vi "Testvi.vi"() -> ()   [LabVIEW 2019]
uses:
  <vilib>/addons/control/pid/pid.llb/PID (DBL).vi
  <vilib>/addons/control/pid/NI_PID_pid.lvlib
panel:
  in  "process variable":dbl format="%.2f"
  in  "setpoint":dbl format="%.2f"
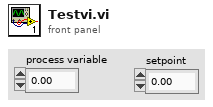
[diagram p1: front panel]
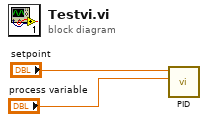
[diagram p0: block diagram]
diagram:
  n1 = call-poly <vilib>:"PID.vi"("process variable"="process variable", "setpoint"="setpoint") -> ()  [unwired: 8 in, 2 out]
